vi "gama1.vi"(9 "Z":dbl, 10 "v0^2":dbl[](array[numeric]), 11 "u0^2":dbl[](array[numeric])) -> (1 "Au below":dbl[](array[numeric]), 2 "Au middle":dbl[](array[numeric]), 3 "gamma1":dbl[](array[numeric]))   [LabVIEW 2021]
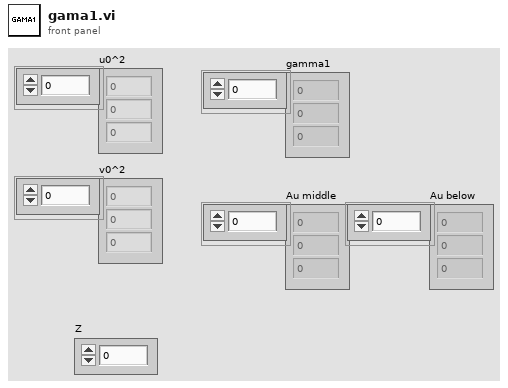
[diagram p1: front panel]
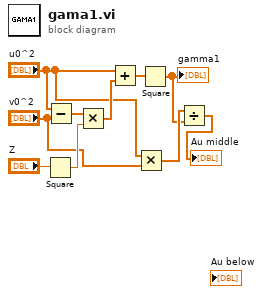
[diagram p0: block diagram]
diagram:
  n1 = Square(x="Z") -> (x^2=w8:dbl)
  n2 = Subtract(x="u0^2", y="v0^2") -> (x-y=w9:dbl[])
  n3 = Multiply(x=w9, y=w8) -> (x*y=w7:dbl[])
  n4 = Add(x="u0^2", y=w7) -> (x+y=w6:dbl[])
  n5 = Multiply(x="u0^2", y="v0^2") -> (x*y=w3:dbl[])
  n6 = Square(x=w6) -> (x^2=w2:dbl[])
  "gamma1" <- w2
  n7 = Divide(x=w3, y=w2) -> (x/y=→"Au middle":dbl[])
